vi "CreateAF-ClassLibrary.vi"(7 "Providername":string="NewActor", 8 "error in (no error)":errorcluster, 10 "ProjectTreePosition(String or Project Item Ref)":variant, 11 "CreateClassData":T1={"ClassName"="A1", "ClassFolder"=path "D:/LabVIEW/2010-T1/A1", "ClassDescription"="", "ClassTemplateOptions"="AF3.0.7_Actor1_GUI_G4_3.0.7", "BaseClass(ProjectStringPath or LvClassFilePath)"=variant(path path "C:/Program Files/National Instruments/LabVIEW 2010/user.lib/_Frameworks/Actor Framework/Actor/Actor.lvclass"), "ExtraCreateParameters"=variant, "FolderSuffix"="_Actor", "ParentInterfaces"=[]}) -> (0 "error out":errorcluster, 2 "TemplateVersionUsed":string, 3 "LVClassLibraryRefnum":refnum<vi>)   [LabVIEW 2020, in "ClassWriterNative.lvclass"]
uses:
  <resource>/Framework/Providers/Open_GDS/ClassProviders/Provider_LvNativeClass/ClassWriterNative_class/ClassWriterNative.lvclass
  <resource>/Framework/Providers/Open_GDS/ClassProviders/Provider_BaseClassInterface/CreateClassData.ctl
  <resource>/Framework/Providers/Open_GDS/ClassProviders/Common/LvClass_class/GDSLvCLass_ClassSettingsType.ctl
  <resource>/Framework/Providers/Open_GDS/ClassProviders/Common/LvClass_class/GDSLvClass_PlugIn.ctl
  <resource>/Framework/Providers/Open_GDS/ClassProviders/Common/LvClass_class/GDSLvClass_PlugInTypes.ctl
  <resource>/Framework/Providers/Open_GDS/ClassProviders/Common/ScriptingFunctions/Scripting_ConnectorPanePatternType.ctl
  <resource>/Framework/Providers/Open_GDS/ClassProviders/Provider_BaseClassInterface/ClassApperanceType.ctl
  <resource>/Framework/Providers/Open_GDS/ClassProviders/Provider_BaseClassInterface/ClassWriter_class/ClassWriter.lvclass
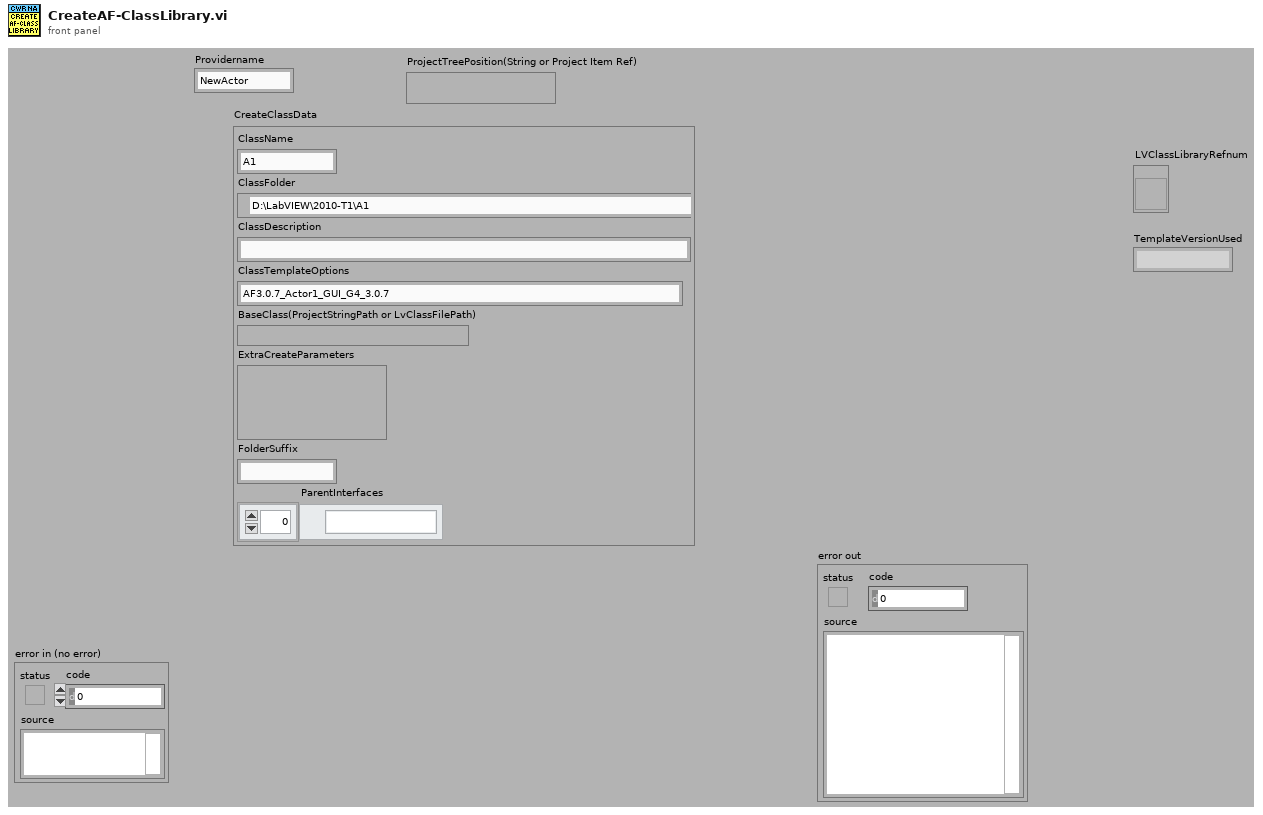
[diagram p1: front panel]
types:
  T1 = typedef "ClassWriter.lvclass/CreateClassData.ctl" = cluster{"ClassName":string, "ClassFolder":path, "ClassDescription":string, "ClassTemplateOptions":string, "BaseClass(ProjectStringPath or LvClassFilePath)":variant, "ExtraCreateParameters":variant, "FolderSuffix":string, "ParentInterfaces":path[]}
  T2 = cluster{"TemplateLib/ClassName":string, "Library":refnum<vi>, "LibraryVIs":refnum<vi>[], "LibraryClasses":refnum<vi>[], "LibraryViNames":string[], "LibraryClassesNames":string[], "TemplateLib/ClassPath":path, "ClassTemplateVersion":string, "App":refnum<vi>, "ProjectRefnum":refnum<vi>, "ProjectItemOwner":refnum<vi>, "VIsRenamed":path[], "ClassesRenamed":path[], "ClassesRootClass":string[], "lvlib":bool, "LibraryVIPaths":path[], "LibraryClassesPaths":path[], "FolderItems":refnum<vi>[], "FolderNames":string[], "AddInheritance":bool[], "LibraryClasses(Path)":path[], "DestroyProjectItemRef":bool}
  T3 = typedef "GDSLvCLass_ClassSettingsType.ctl" = cluster{"ClassProviderName":string, "ClassTemplateUsed":string, "ClassTemplateVersion":string, "ClassDescription":string, "PlugIns":T4[], "ConnectorPanePattern":string}
  T4 = typedef "GDSLvClass_PlugIn.ctl" = cluster{"Type":T5, "ID":string, "Version":string, "Path":path, "Name":string, "Data":variant}
  T5 = typedef "GDSLvClass_PlugInTypes.ctl" = enum16{"DesignPattern", "MethodTypes"}
  T6 = typedef "ClassApperanceType.ctl" = enum16{"Class", "AF-MessageClass", "Interface"}
  T7 = cluster{"LibraryIcon":string, "HeaderRows(1)":u8}
  T8 = cluster{"Major":u16, "Minor":u16, "Fix":u16, "Build":u16}
  T9 = typedef "AF_SettingsType.ctl" = cluster{"MessageFolderName":string}
  T10 = typedef "Scripting_ConnectorPanePatternType.ctl" = u16
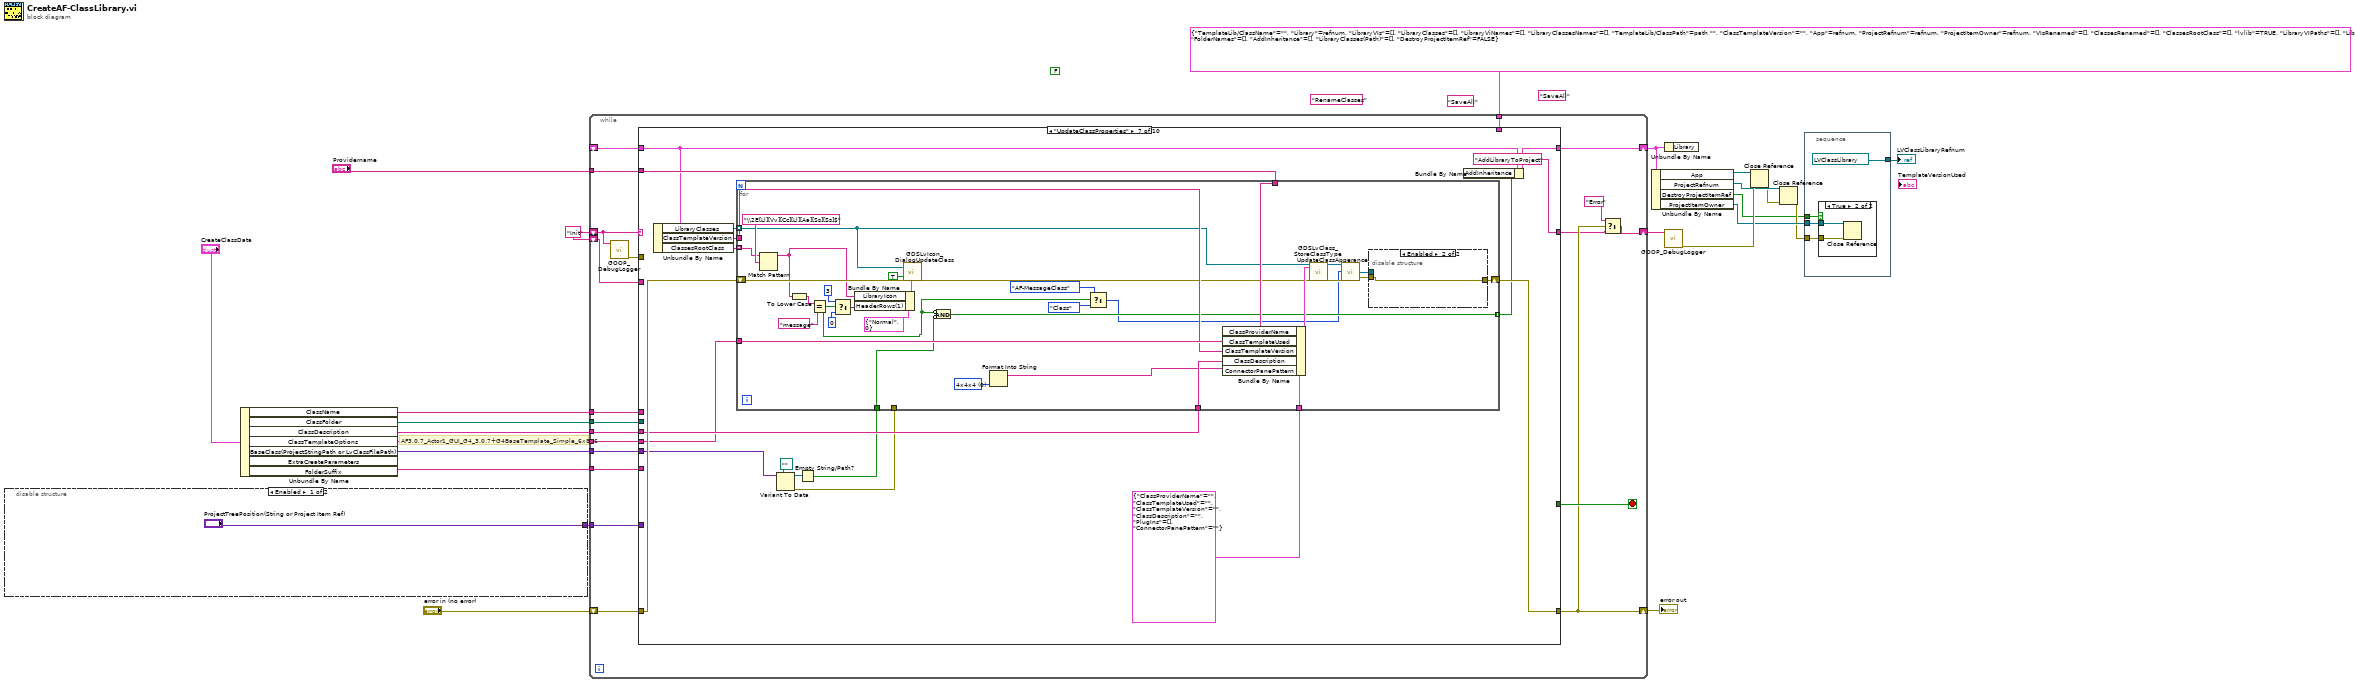
[diagram p0: block diagram]
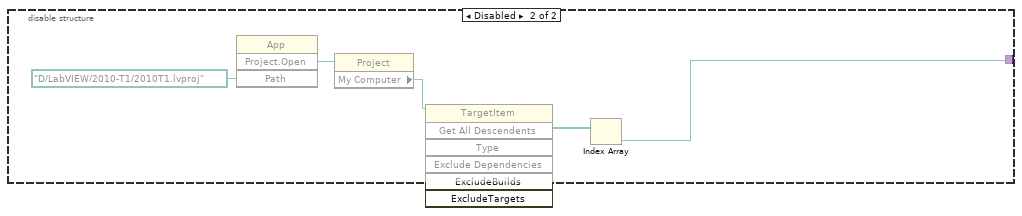
[diagram p3: hidden frame]
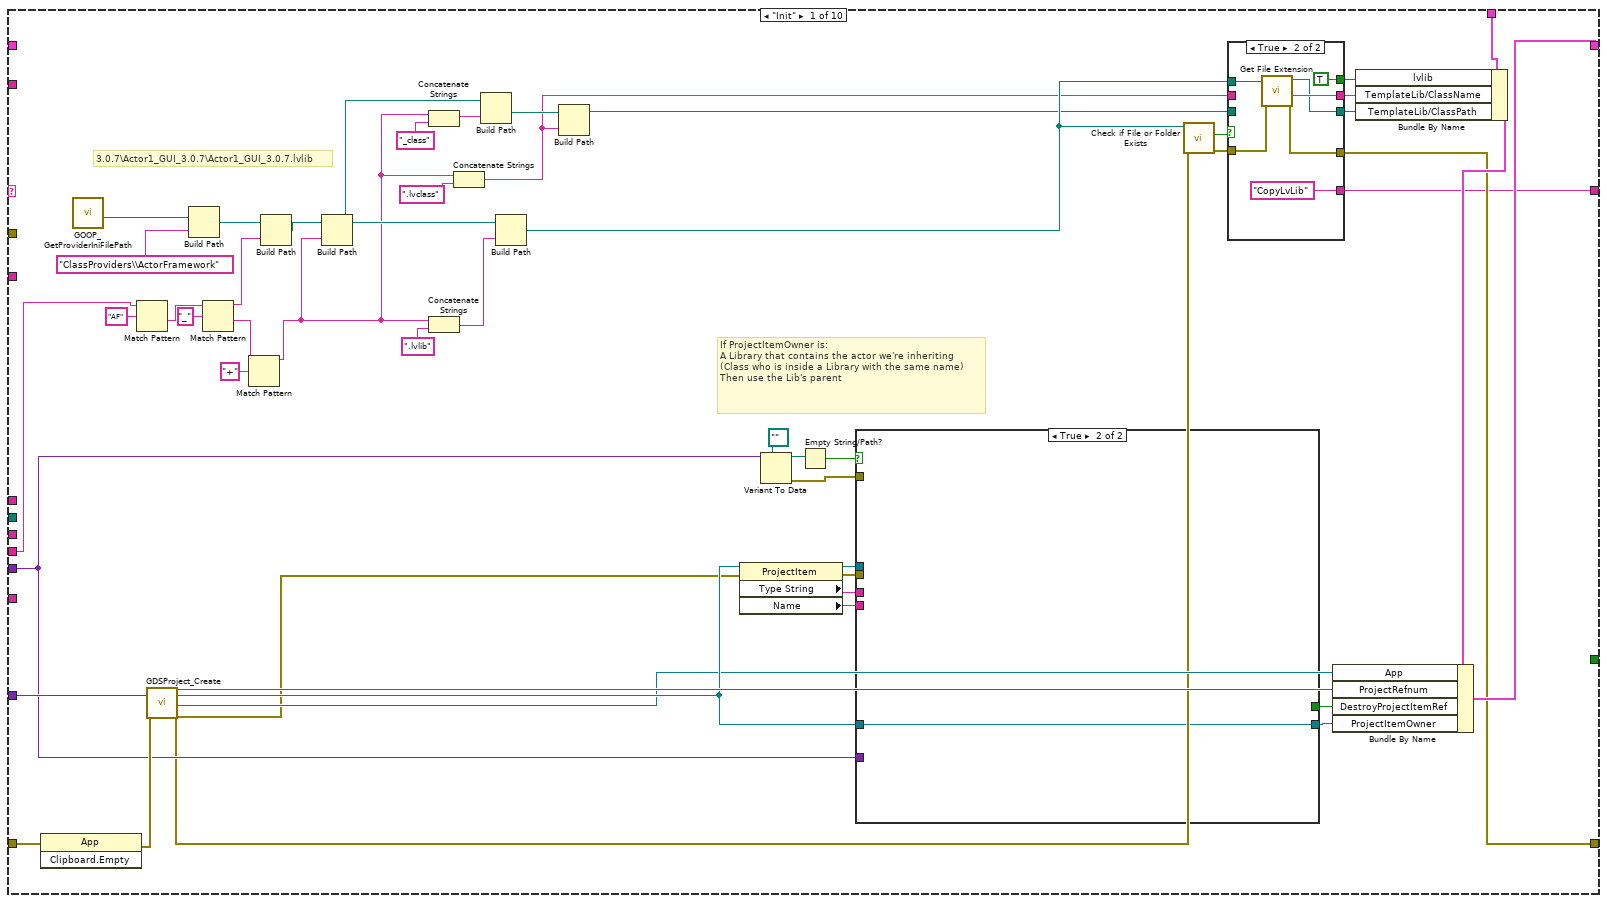
[diagram p4: hidden frame]
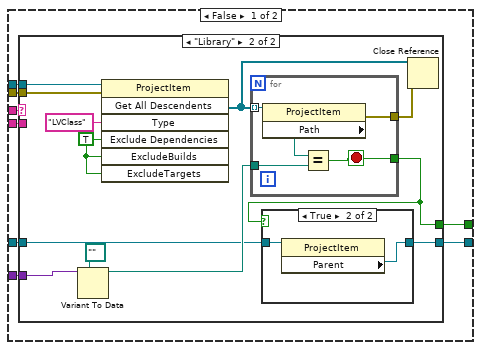
[diagram p5: hidden frame]
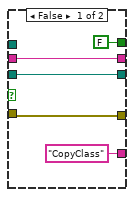
[diagram p8: hidden frame]
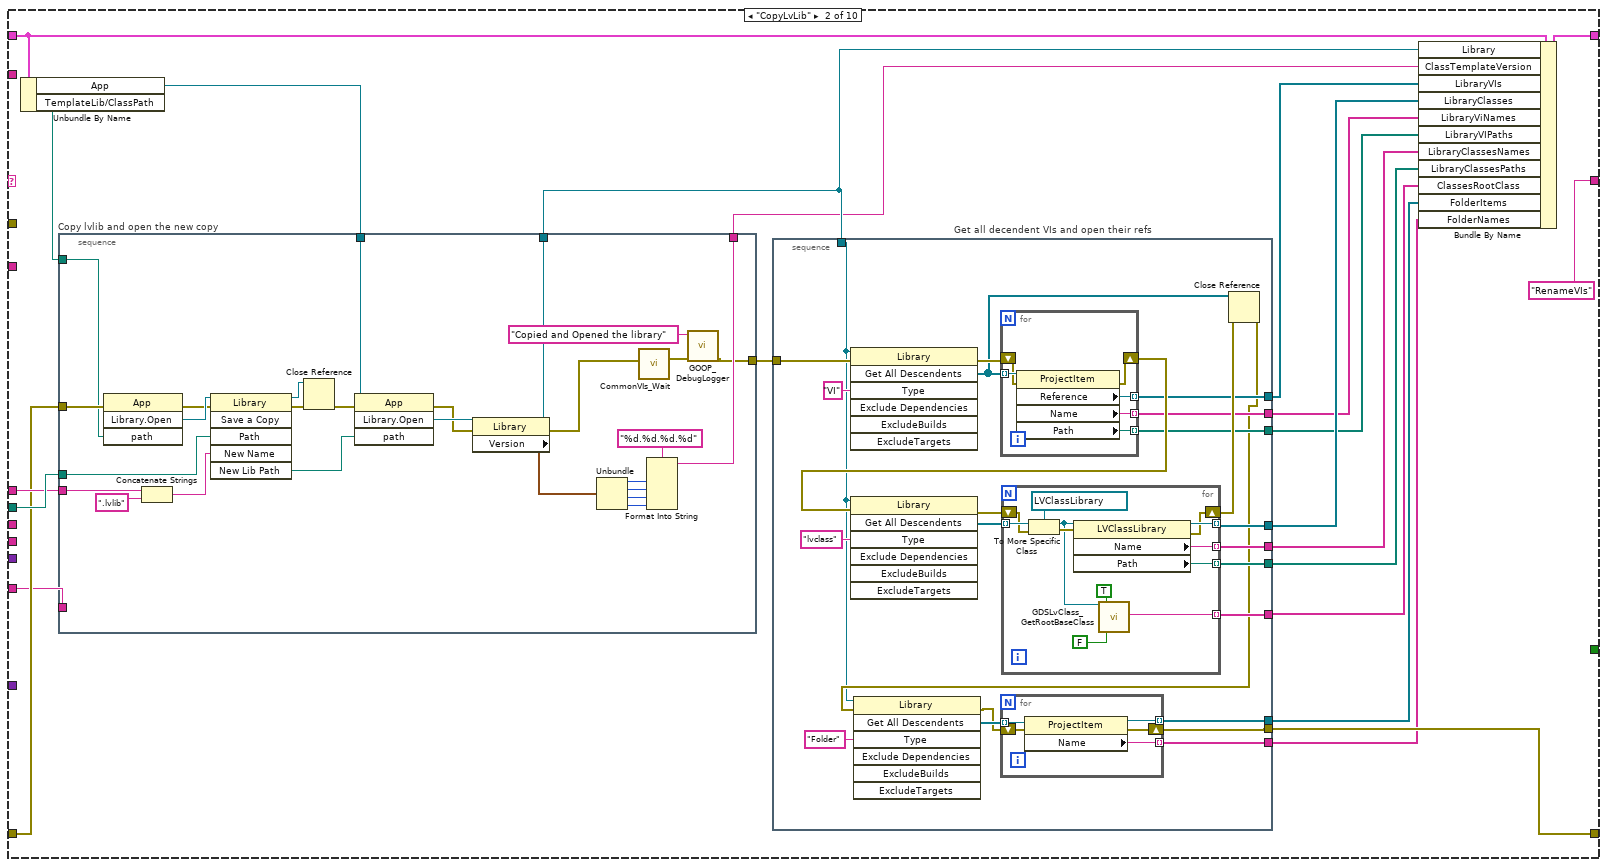
[diagram p9: hidden frame]
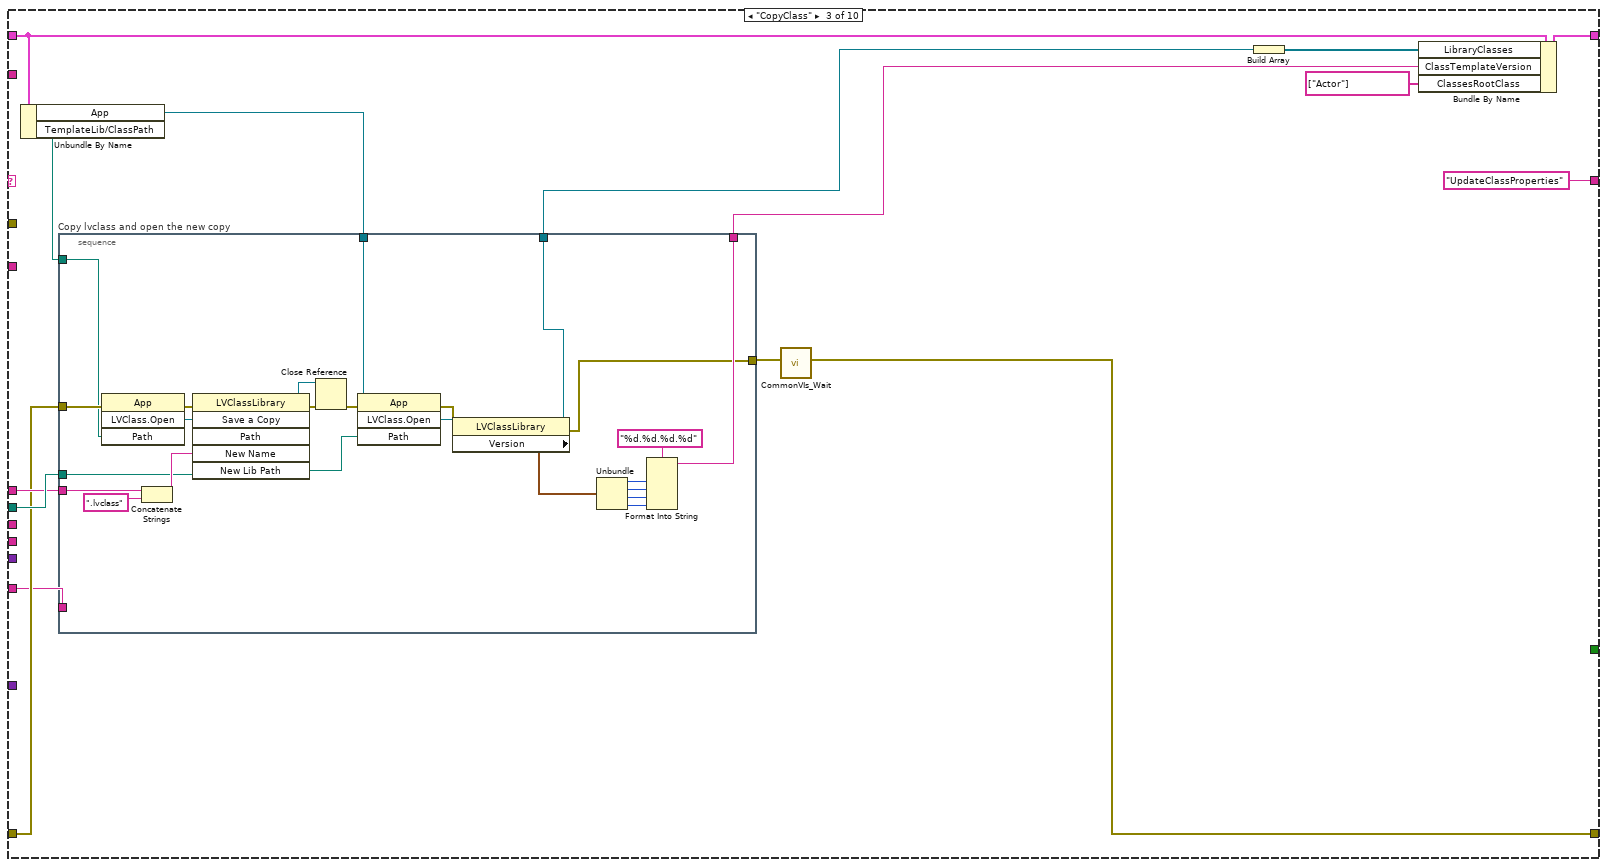
[diagram p10: hidden frame]
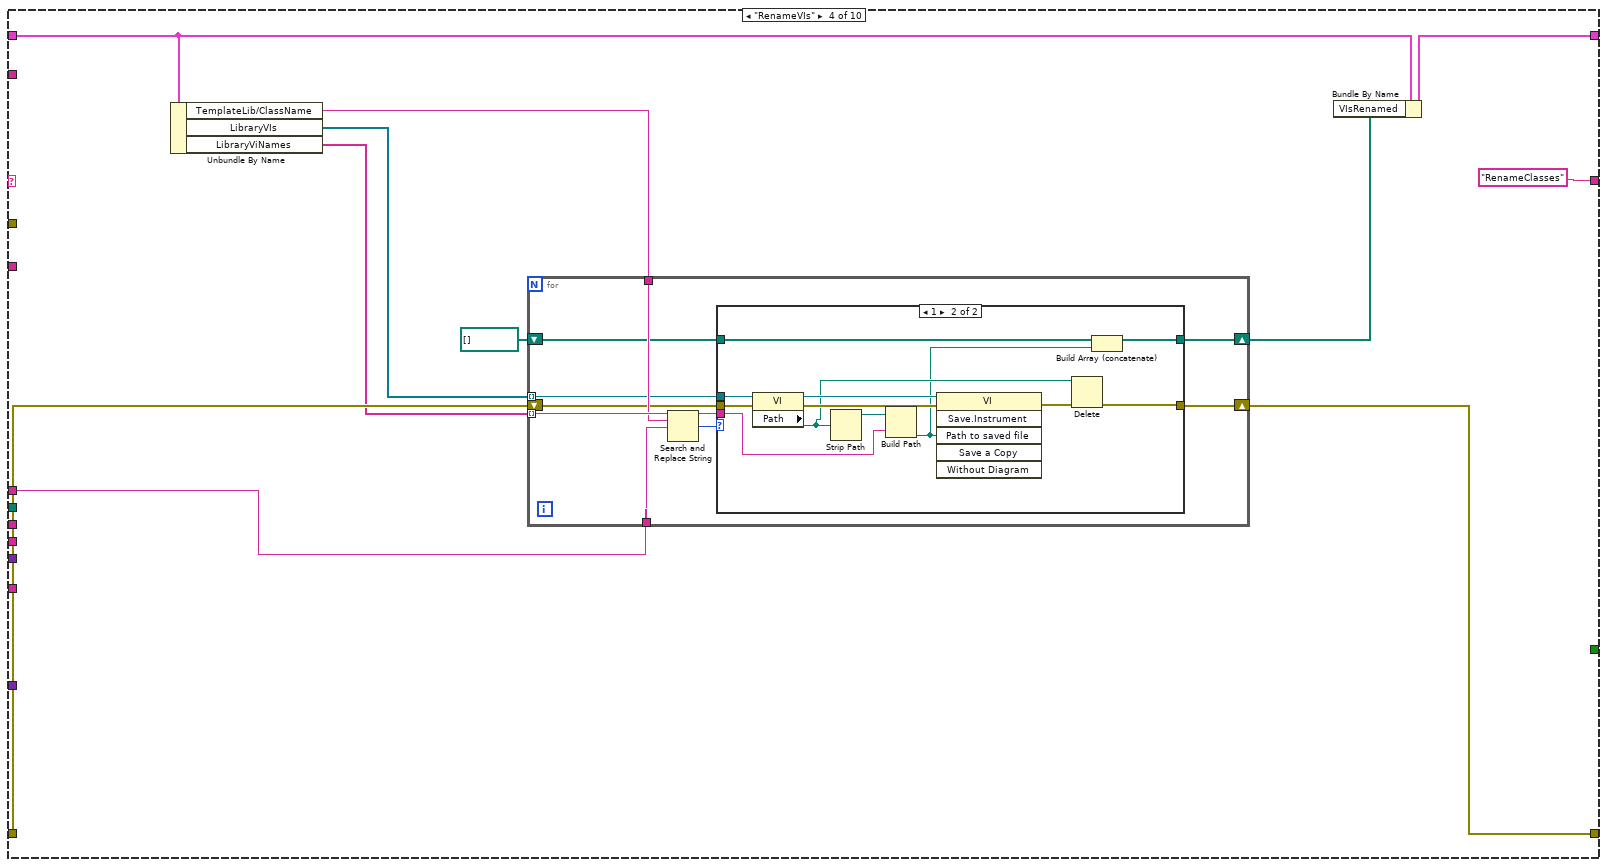
[diagram p11: hidden frame]
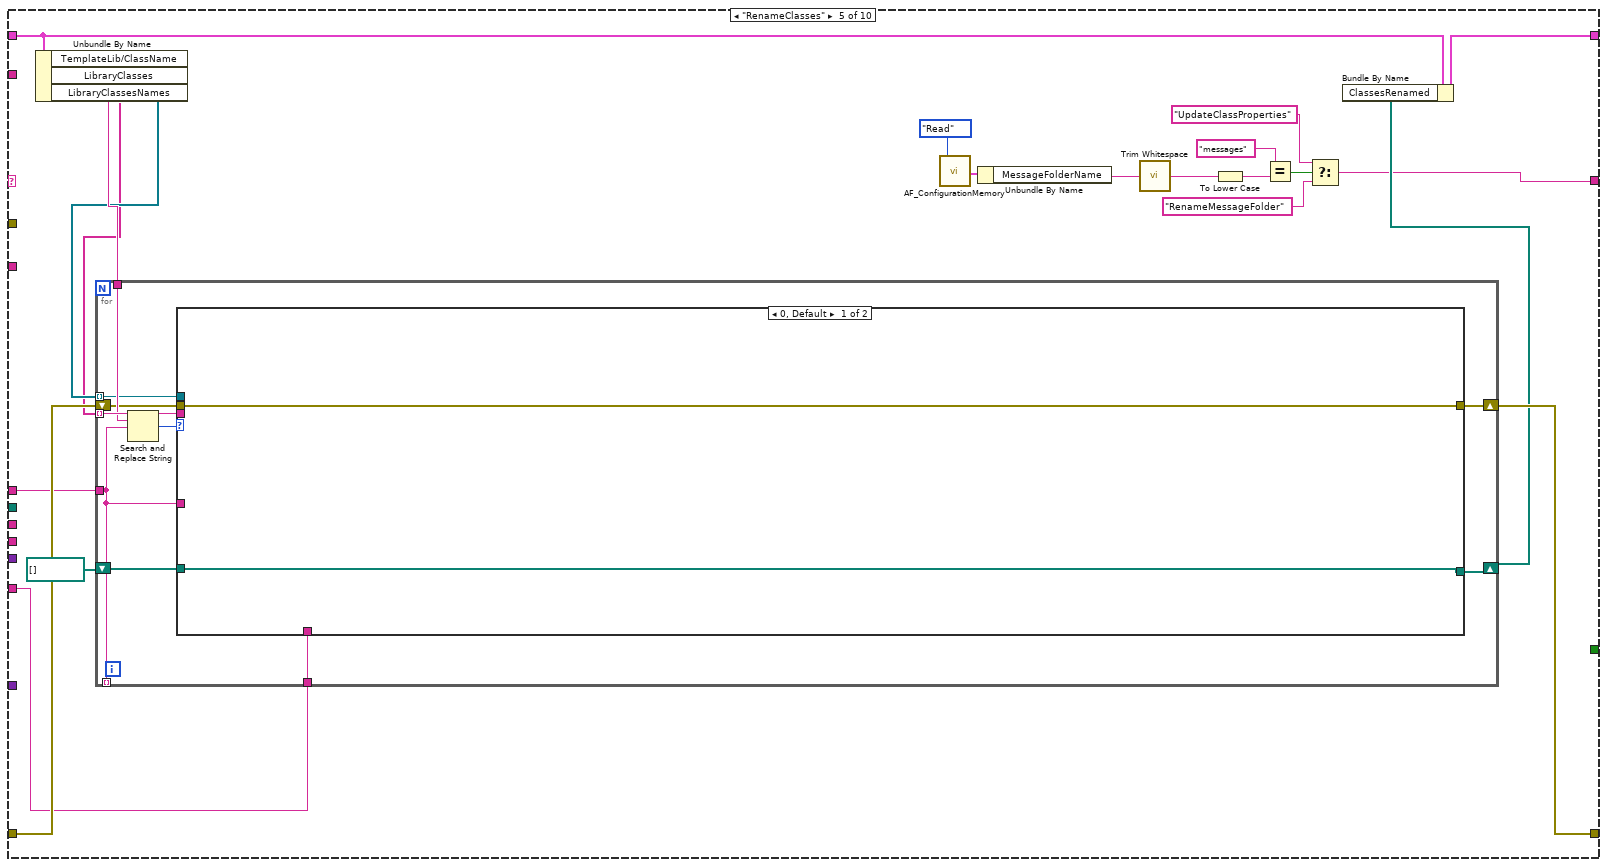
[diagram p13: hidden frame]
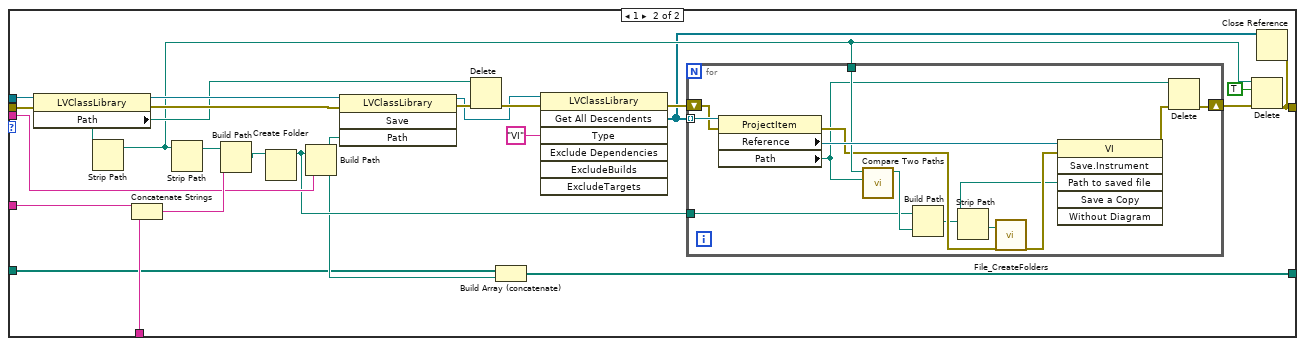
[diagram p14: hidden frame]
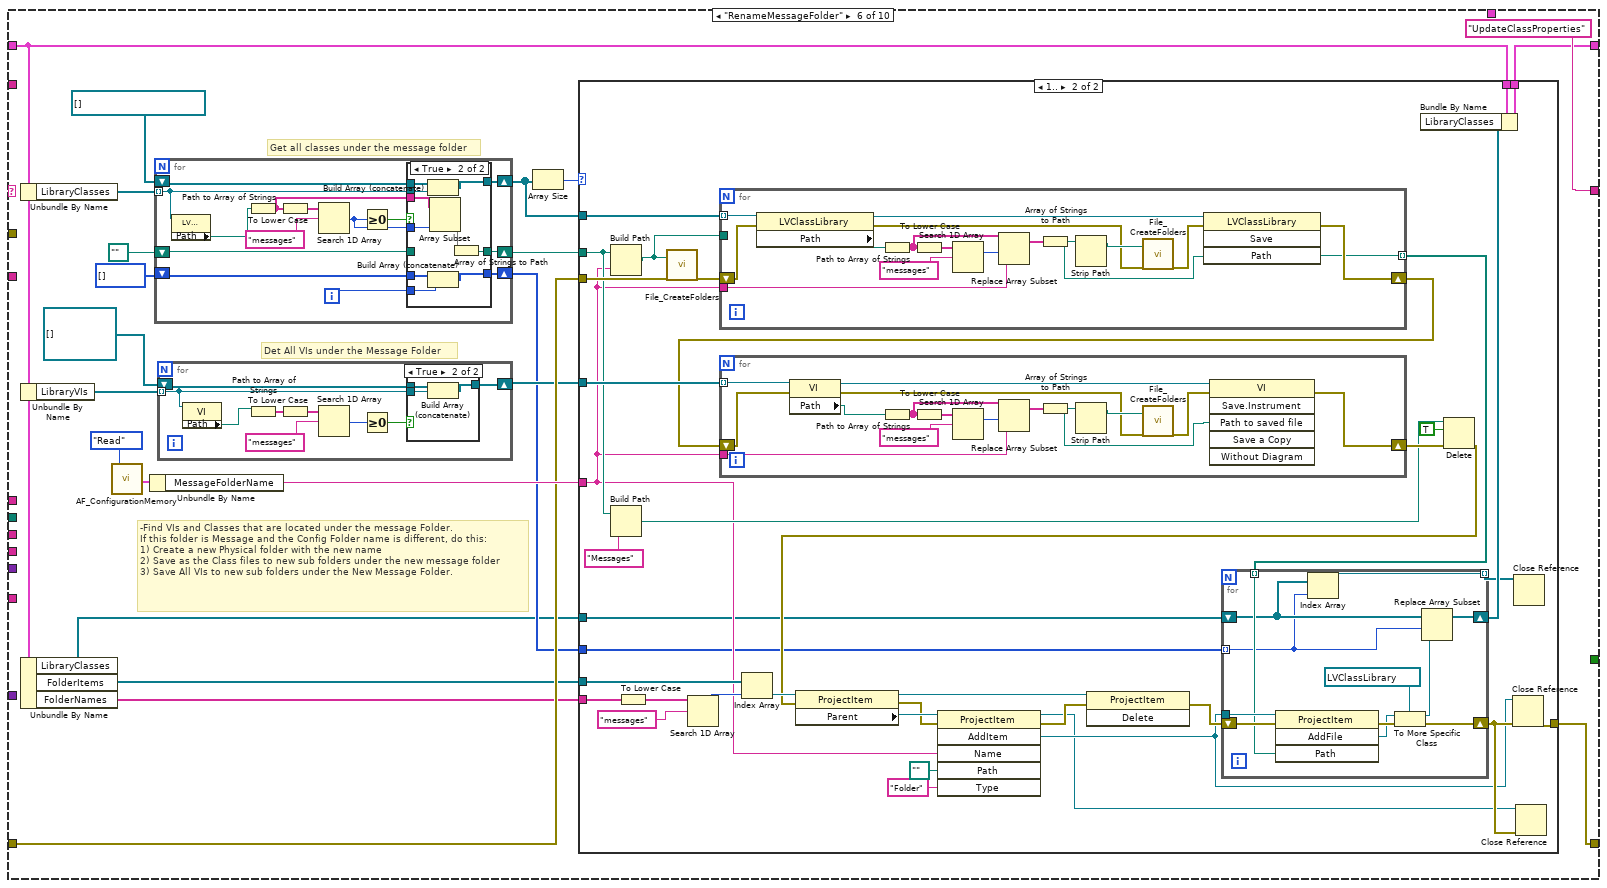
[diagram p15: hidden frame]
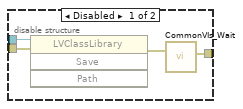
[diagram p19: hidden frame]
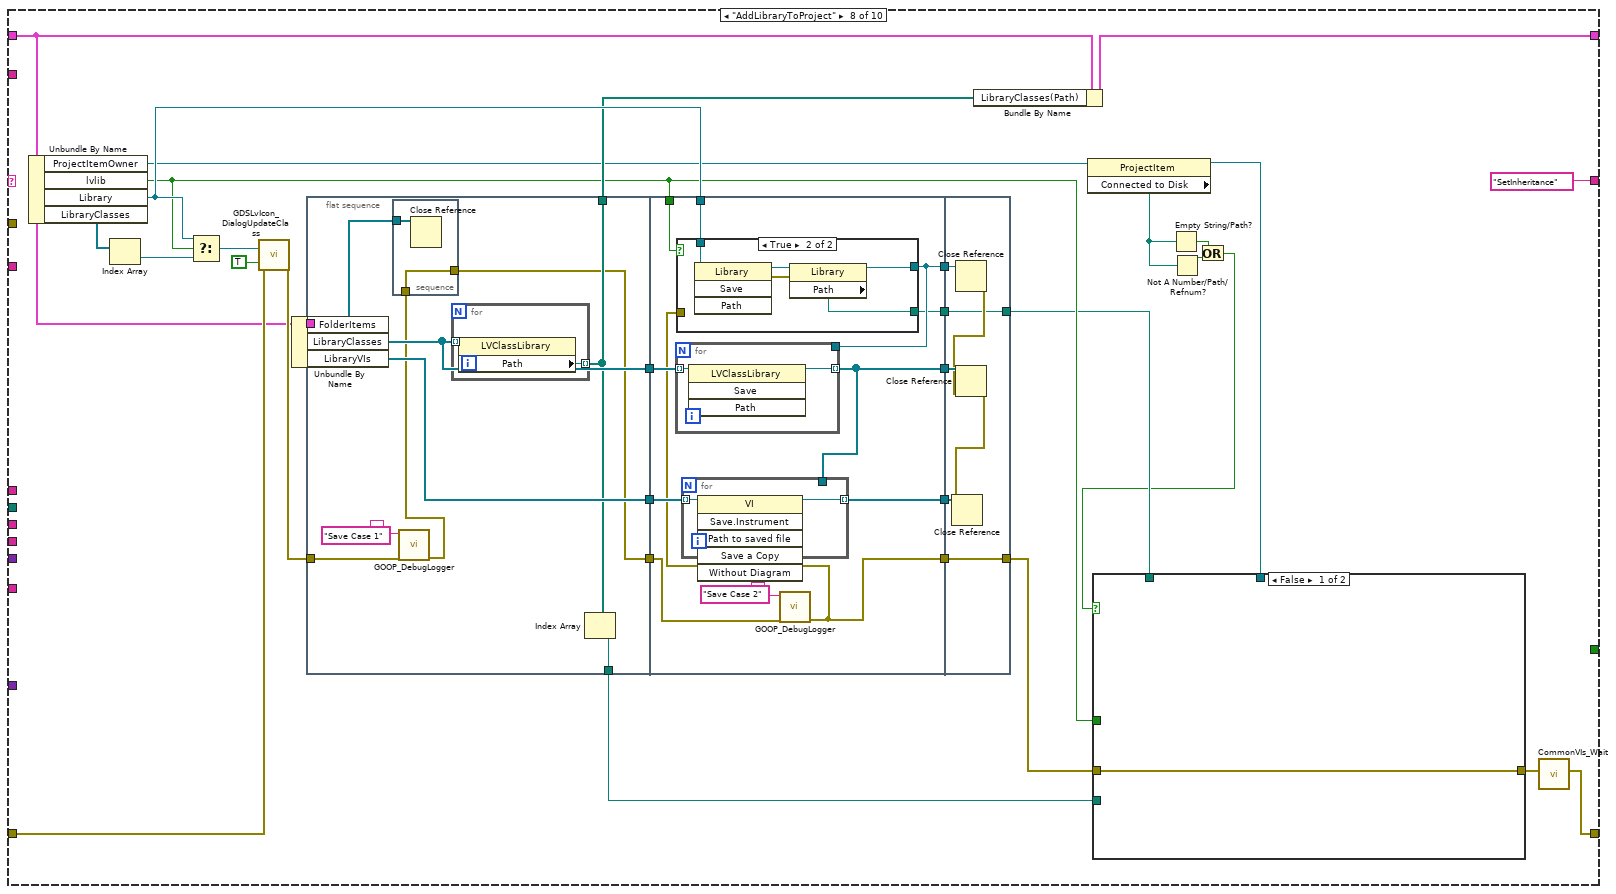
[diagram p20: hidden frame]
diagram:
  (unwired) FALSE ("LimitToSpecificProviderTypeOfSameType(True)")
  (unwired) "RenameClasses" ("Name")
  (unwired) "SaveAll" ("Name")
  (unwired) "SaveAll" ("Name")
  w1 = "Init" ("string")
  # "AF3.0.7_Actor1_GUI_G4_3.0.7+G4BaseTemplate_Simple_6x8x6"
  n1 = disable-structure shown="Enabled" {
    disable-tunnel: ["ProjectTreePosition(String or Project Item Ref)" w25] -> w13
    frame Enabled {
    }
    frame Disabled {
      n2 = invoke class="App" method="Project.Open"("Path"=path "D:/LabVIEW/2010-T1/2010T1.lvproj") -> ("Project:Open"=w28:refnum<vi>)  [unwired: 3 in, 3 out]
      n3 = property class="Project"(reference=w28) -> ("My Computer"=w26:refnum<vi>)  [unwired: 1 in, 2 out]
      n4 = invoke class="TargetItem" method="Get All Descendents"(reference=w26) -> ("All Descendents"=w27:refnum<vi>[])  [unwired: 6 in, 6 out]
      n5 = Index Array(array=w27) -> (element=w25:refnum<vi>)  [unwired: 1 in]
    }
  }
  n6 = Unbundle By Name("CreateClassData") -> ("ClassName"=w20:string, "ClassFolder"=w17:path, "ClassDescription"=w14:string, "ClassTemplateOptions"=w16:string, "BaseClass(ProjectStringPath or LvClassFilePath)"=w11:variant, "FolderSuffix"=w19:string)  [unwired: 1 out]
  n7 = while {
    tunnel: w17 -> [w49]
    tunnel: w20 -> [w48]
    tunnel: w19 -> [w46]
    shift-right: [w31] -> w9
    shift-left: w1 -> [w36]
    shift-right: [w44] -> w12
    shift-left: _ -> [w43]
    tunnel: T2 {"TemplateLib/ClassName"="", "Library"=refnum, "LibraryVIs"=[], "LibraryClasses"=[], "LibraryViNames"=[], "LibraryClassesNames"=[], "TemplateLib/ClassPath"=path "", "ClassTemplateVersion"="", "App"=refnum, "ProjectRefnum"=refnum, "ProjectItemOwner"=refnum, "VIsRenamed"=[], "ClassesRenamed"=[], "ClassesRootClass"=[], "lvlib"=TRUE, "LibraryVIPaths"=[], "LibraryClassesPaths"=[], "FolderItems"=[], "FolderNames"=[], "AddInheritance"=[], "LibraryClasses(Path)"=[], "DestroyProjectItemRef"=FALSE} -> [w45]
    shift-right: [w33] -> w18
    shift-left: "error in (no error)" -> [w47]
    tunnel: w16 -> [w41]
    tunnel: "Providername" -> [w40]
    tunnel: w14 -> [w39]
    tunnel: w13 -> [w38]
    tunnel: w11 -> [w37]
    shift-left: w1 -> [w34]
    stop <- w42 stop-if-true
    n8 = call <resource>:"GOOP_DebugLogger.vi"("State"=w36) -> ("error out"=w35:errorcluster)  [unwired: 8 in, 2 out]
    n9 = case shown="\"UpdateClassProperties\"" w36 {
      tunnel: w49 -> [_ w163 w252 _ _ _ _ _ _ _]
      tunnel: w48 -> [_ w162 w251 w284 w328 _ _ _ _ _]
      tunnel: [w78 w160 w239 w285 w326 w389 w535 w597 w686 w708] -> w33
      tunnel: w47 -> [w65 w159 w250 w286 w332 w393 w542 w612 w687 w709]
      tunnel: w46 -> [_ w158 w249 _ w327 _ _ _ _ _]
      tunnel: w45 -> [w99 _ _ _ _ _ _ _ _ _]
      tunnel: [w85 w152 w247 w278 w323 w384 w532 w593 w685 w706] -> w44
      tunnel: [w75 "RenameVIs" ("Name") "UpdateClassProperties" ("filename without extension") "RenameClasses" ("Name") w313 "UpdateClassProperties" ("filename without extension") "AddLibraryToProject" ("Name") "SetInheritance" ("Name") "Exit" ("Name") "Exit" ("Name")] -> w32
      tunnel: w43 -> [_ w149 w245 w279 w324 w385 w533 w594 w685 w706]
      tunnel: [_ _ _ _ _ _ _ _ _ TRUE] -> w42
      tunnel: w41 -> [w94 _ _ _ _ _ w538 _ _ _]
      tunnel: w40 -> [_ _ _ _ _ _ w541 _ _ _]
      tunnel: w39 -> [_ _ _ _ _ _ w540 _ _ _]
      tunnel: w38 -> [w83 _ _ _ _ _ _ _ _ _]
      tunnel: w37 -> [w56 _ _ _ _ _ w529 _ w683 _]
      tunnel: w35 -> [_ _ _ _ _ _ _ _ _ _]
      tunnel: w34 -> [_ _ _ _ _ _ _ _ _ w707]
      frame "Init" {
        # "If ProjectItemOwner is:\nA Library that contains the actor we're inheriting\n(Class who is inside a Library with the same name)\nThen use the Lib's parent"
        # "3.0.7\\Actor1_GUI_3.0.7\\Actor1_GUI_3.0.7.lvlib"
        n10 = invoke class="App" method="Clipboard.Empty"(error in=w65) -> (error out=w64:errorcluster)  [unwired: 2 in, 2 out]
        n11 = call <resource>:"GOOP_GetProviderIniFilePath.vi"() -> ("ProviderMainFolder"=w96:path)  [unwired: 10 in, 1 out]
        n12 = Match Pattern(string=w94, regular expression="AF") -> (after substring=w92:string)  [unwired: 1 in, 3 out]
        n13 = call <resource>:"GDSProject_Create.vi"("ProjectTreePosition(String or Project Item Ref)"=w83, "error in (no error)"=w64) -> ("Project Refnum"=w86:refnum<vi>, "Project Item"=w59:refnum<vi>, "App"=w51:refnum<vi>, "error out"=w50:errorcluster)  [unwired: 13 in, 1 out]
        n14 = Build Path(base path=w96, name or relative path="ClassProviders\\ActorFramework") -> (appended path=w97:path)
        n15 = Match Pattern(string=w92, regular expression="_") -> (before substring=w90:string, after substring=w82:string)  [unwired: 1 in, 2 out]
        n16 = Match Pattern(string=w82, regular expression="+") -> (before substring=w70:string)  [unwired: 1 in, 3 out]
        n17 = Build Path(base path=w97, name or relative path=w90) -> (appended path=w89:path)
        n18 = Build Path(base path=w89, name or relative path=w70) -> (appended path=w74:path)
        n19 = Concatenate Strings(w70, "_class" ("string")) -> (w72:string)
        n20 = Concatenate Strings(w70, ".lvlib" ("string")) -> (w87:string)
        n21 = Concatenate Strings(w70, ".lvclass" ("string")) -> (w68:string)
        n22 = Build Path(base path=w74, name or relative path=w72) -> (appended path=w71:path)
        n23 = Build Path(base path=w74, name or relative path=w87) -> (appended path=w80:path)
        n24 = Build Path(base path=w71, name or relative path=w68) -> (appended path=w67:path)
        n25 = property class="ProjectItem"(reference=w59, error in=w50) -> (reference out=w61:refnum<vi>, error out=w60:errorcluster, "Type String"=w63:string, "Name"=w62:string)
        n26 = Variant To Data(type=path "" ("Path"), Variant=w56) -> (data=w54:path, error out=w52:errorcluster)  [unwired: 1 in]
        n27 = Empty String/Path?(string/path=w54) -> (empty?=w53:bool)
        n28 = case shown="True" w53 {
          tunnel: w63 -> [w107 _]
          tunnel: w62 -> [w106 _]
          tunnel: w61 -> [w105 _]
          tunnel: w60 -> [w104 _]
          tunnel: w56 -> [w103 _]
          tunnel: w59 -> [w102 w129]
          tunnel: [w101 w129] -> w58
          tunnel: [w100 _] -> w57
          tunnel: w52 -> [_ _]
          frame False {
            n29 = case shown="\"Library\"" w107 {
              tunnel: w106 -> [_ _]
              tunnel: w105 -> [_ w120]
              tunnel: w104 -> [_ w119]
              tunnel: w103 -> [_ w116]
              tunnel: w102 -> [w108 w113]
              tunnel: [w108 w112] -> w101
              tunnel: [_ w111] -> w100
              frame "False", Default {
              }
              frame "Library" {
                w117 = TRUE ("ExcludeDependencies")
                n30 = Variant To Data(type=path "" ("Path"), Variant=w116) -> (data=w115:path)  [unwired: 1 in, 1 out]
                n31 = invoke class="ProjectItem" method="Get All Descendents"(reference=w120, error in=w119, "Type"="LVClass", "Exclude Dependencies"=w117, "ExcludeBuilds"=w117, "ExcludeTargets"=w117) -> ("All Descendents"=w109:refnum<vi>[])  [unwired: 1 in, 6 out]
                n32 = for {
                  tunnel: w109 -> [w128] mode=indexing
                  tunnel: w115 -> [w126]
                  tunnel: [w125] -> w111
                  tunnel: [w124] -> w110
                  stop <- w125 stop-if-true
                  n33 = property class="ProjectItem"(reference=w128) -> (error out=w124:errorcluster, "Path"=w127:path)  [unwired: 1 in, 1 out]
                  n34 = Equal?(x=w127, y=w126) -> (x = y?=w125:bool)
                }
                n35 = case shown="True" w111 {
                  tunnel: w113 -> [w121 w123]
                  tunnel: [w121 w122] -> w112
                  frame False {
                  }
                  frame True {
                    n36 = property class="ProjectItem"(reference=w123) -> ("Parent"=w122:refnum<vi>)  [unwired: 1 in, 2 out]
                  }
                }
                n37 = Close Reference(reference=w109, error in (no error)=w110) -> ()  [unwired: 1 out]
              }
            }
          }
          frame True {
          }
        }
        n38 = call <vilib>:"Check if File or Folder Exists.vi"("error in (no error)"=w50, "path"=w80) -> ("error out"=w79:errorcluster, "file or folder exists?"=w77:bool)  [unwired: 7 in, 1 out]
        n39 = case shown="True" w77 {
          tunnel: [w132 w141] -> w98
          tunnel: w80 -> [_ w140]
          tunnel: w79 -> [w134 w139]
          tunnel: [w134 w138] -> w78
          tunnel: [w131 w137] -> w76
          tunnel: ["CopyClass" ("Name") "CopyLvLib" ("Name")] -> w75
          tunnel: w68 -> [w132 _]
          tunnel: w67 -> [w131 _]
          tunnel: [FALSE TRUE] -> w66
          frame False {
          }
          frame True {
            n40 = call <vilib>:"Get File Extension.vi"("error in (no error)"=w139, "file"=w140) -> ("error out"=w138:errorcluster, "filename without extension"=w141:string, "dup file"=w137:path)  [unwired: 5 in, 2 out]
          }
        }
        n41 = Bundle By Name(cluster=w99, "lvlib"=w66, "TemplateLib/ClassName"=w98, "TemplateLib/ClassPath"=w76) -> (w84:T2)
        n42 = Bundle By Name(cluster=w84, "App"=w51, "ProjectRefnum"=w86, "DestroyProjectItemRef"=w57, "ProjectItemOwner"=w58) -> (w85:T2)
      }
      frame "CopyLvLib" {
        n43 = Unbundle By Name(w149) -> ("App"=w142:refnum<vi>, "TemplateLib/ClassPath"=w150:path)
        n44 = stacked-sequence "Copy lvlib and open the new copy" {
          tunnel: w163 -> [w226]
          tunnel: w158 -> [_]
          tunnel: w162 -> [w233]
          tunnel: [w217] -> w157
          tunnel: [w213] -> w161
          tunnel: w159 -> [w228]
          tunnel: w150 -> [w227]
          tunnel: [w216] -> w148
          tunnel: w142 -> [w211]
          frame #0 {
            n45 = invoke class="App" method="Library.Open"(error in=w228, "path"=w227) -> (error out=w235:errorcluster, "Open Library"=w237:refnum<vi>)  [unwired: 2 in, 2 out]
            n46 = Concatenate Strings(w233, ".lvlib" ("string")) -> (w236:string)
            n47 = invoke class="Library" method="Save a Copy"(reference=w237, error in=w235, "Path"=w226, "New Name"=w236) -> (reference out=w230:refnum<vi>, error out=w232:errorcluster, "New Lib Path"=w229:path)  [unwired: 2 in, 3 out]
            n48 = Close Reference(reference=w230, error in (no error)=w232) -> (error out=w231:errorcluster)
            n49 = invoke class="App" method="Library.Open"(reference=w211, error in=w231, "path"=w229) -> (error out=w218:errorcluster, "Open Library"=w219:refnum<vi>)  [unwired: 1 in, 2 out]
            n50 = property class="Library"(reference=w219, error in=w218) -> (reference out=w217:refnum<vi>, error out=w215:errorcluster, "Version"=w220:T8)
            n51 = Unbundle(w220) -> ("Major"=w222:u16, "Minor"=w223:u16, "Fix"=w224:u16, "Build"=w225:u16)
            n52 = call <resource>:"CommonVIs_Wait.vi"("error in"=w215) -> ("error out"=w214:errorcluster)  [unwired: 9 in]
            n53 = Format Into String(format string="%d.%d.%d.%d", w222, w223, w224, w225) -> (resulting string=w216:string)  [unwired: 2 in, 1 out]
            n54 = call <resource>:"GOOP_DebugLogger.vi"("error in (no error)"=w214, "State"="Copied and Opened the library") -> ("error out"=w213:errorcluster)  [unwired: 7 in, 2 out]
          }
        }
        n55 = stacked-sequence "Get all decendent VIs and open their refs" {
          tunnel: w157 -> [w170]
          tunnel: w161 -> [w187]
          tunnel: [w166] -> w160
          tunnel: [w178] -> w156
          tunnel: [w177] -> w153
          tunnel: [w176] -> w154
          tunnel: [w175] -> w155
          tunnel: [w174] -> w147
          tunnel: [w173] -> w146
          tunnel: [w172] -> w145
          tunnel: [w167] -> w144
          tunnel: [w164] -> w143
          frame #0 {
            n56 = invoke class="Library" method="Get All Descendents"(reference=w170, error in=w187, "Type"="VI") -> (error out=w185:errorcluster, "All Descendents"=w184:refnum<vi>[])  [unwired: 4 in, 5 out]
            n57 = for {
              tunnel: w184 -> [w210] mode=indexing
              shift-right: [w208] -> w182
              shift-left: w185 -> [w209]
              tunnel: [w207] -> w178 mode=indexing
              tunnel: [w206] -> w176 mode=indexing
              tunnel: [w205] -> w173 mode=indexing
              n58 = property class="ProjectItem"(reference=w210, error in=w209) -> (error out=w208:errorcluster, "Reference"=w207:refnum<vi>, "Name"=w206:string, "Path"=w205:path)  [unwired: 1 out]
            }
            n59 = invoke class="Library" method="Get All Descendents"(reference=w170, error in=w182, "Type"="lvclass") -> (error out=w180:errorcluster, "All Descendents"=w181:refnum<vi>[])  [unwired: 4 in, 5 out]
            n60 = for {
              tunnel: w181 -> [w204] mode=indexing
              shift-right: [w200] -> w179
              shift-left: w180 -> [w202]
              tunnel: [w201] -> w175 mode=indexing
              tunnel: [w198] -> w177 mode=indexing
              tunnel: [w194] -> w174 mode=indexing
              tunnel: [w193] -> w172 mode=indexing
              n61 = To More Specific Class(target class=refnum<vi> refnum ("Library"), reference=w204, error in=w202) -> (specific class reference=w197:refnum<vi>, error out=w199:errorcluster)
              n62 = property class="LVClassLibrary"(reference=w197, error in=w199) -> (reference out=w201:refnum<vi>, error out=w200:errorcluster, "Name"=w198:string, "Path"=w193:path)
              n63 = call <resource>:"GDSLvClass_GetRootBaseClass.vi"("ViRef/Path,LvClassRef/Path"=w197, "Don'tOpenReference"=TRUE, "LimitToSpecificProviderTypeOfSameType(True)"=FALSE) -> ("ClassName"=w194:string)  [unwired: 10 in, 6 out]
            }
            n64 = Close Reference(reference=w184, error in (no error)=w179) -> (error out=w171:errorcluster)
            n65 = invoke class="Library" method="Get All Descendents"(reference=w170, error in=w171, "Type"="Folder") -> (error out=w165:errorcluster, "All Descendents"=w168:refnum<vi>[])  [unwired: 4 in, 5 out]
            n66 = for {
              tunnel: w168 -> [w192] mode=indexing
              tunnel: [w191] -> w167 mode=indexing
              shift-right: [w190] -> w166
              shift-left: w165 -> [w189]
              tunnel: [w188] -> w164 mode=indexing
              n67 = property class="ProjectItem"(reference=w192, error in=w189) -> (reference out=w191:refnum<vi>, error out=w190:errorcluster, "Name"=w188:string)
            }
          }
        }
        n68 = Bundle By Name(cluster=w149, "Library"=w157, "ClassTemplateVersion"=w148, "LibraryVIs"=w156, "LibraryClasses"=w155, "LibraryViNames"=w154, "LibraryVIPaths"=w146, "LibraryClassesNames"=w153, "LibraryClassesPaths"=w145, "ClassesRootClass"=w147, "FolderItems"=w144, "FolderNames"=w143) -> (w152:T2)
      }
      frame "CopyClass" {
        n69 = Unbundle By Name(w245) -> ("App"=w238:refnum<vi>, "TemplateLib/ClassPath"=w246:path)
        n70 = stacked-sequence "Copy lvclass and open the new copy" {
          tunnel: w252 -> [w265]
          tunnel: w249 -> [_]
          tunnel: w251 -> [w272]
          tunnel: [w256] -> w248
          tunnel: [w254] -> w240
          tunnel: w250 -> [w267]
          tunnel: w246 -> [w266]
          tunnel: [w255] -> w244
          tunnel: w238 -> [w253]
          frame #0 {
            n71 = invoke class="App" method="LVClass.Open"(error in=w267, "Path"=w266) -> (error out=w274:errorcluster, "LVClass.Open"=w276:refnum<vi>)  [unwired: 2 in, 2 out]
            n72 = Concatenate Strings(w272, ".lvclass" ("string")) -> (w275:string)
            n73 = invoke class="LVClassLibrary" method="Save a Copy"(reference=w276, error in=w274, "Path"=w265, "New Name"=w275) -> (reference out=w269:refnum<vi>, error out=w271:errorcluster, "New Lib Path"=w268:path)  [unwired: 2 in, 3 out]
            n74 = Close Reference(reference=w269, error in (no error)=w271) -> (error out=w270:errorcluster)
            n75 = invoke class="App" method="LVClass.Open"(reference=w253, error in=w270, "Path"=w268) -> (error out=w257:errorcluster, "LVClass.Open"=w258:refnum<vi>)  [unwired: 1 in, 2 out]
            n76 = property class="LVClassLibrary"(reference=w258, error in=w257) -> (reference out=w256:refnum<vi>, error out=w254:errorcluster, "Version"=w259:T8)
            n77 = Unbundle(w259) -> ("Major"=w261:u16, "Minor"=w262:u16, "Fix"=w263:u16, "Build"=w264:u16)
            n78 = Format Into String(format string="%d.%d.%d.%d", w261, w262, w263, w264) -> (resulting string=w255:string)  [unwired: 2 in, 1 out]
          }
        }
        n79 = call <resource>:"CommonVIs_Wait.vi"("error in"=w240) -> ("error out"=w239:errorcluster)  [unwired: 9 in]
        n80 = Build Array(w248) -> (w242:refnum<vi>[])
        n81 = Bundle By Name(cluster=w245, "LibraryClasses"=w242, "ClassTemplateVersion"=w244, "ClassesRootClass"=string[] ["Actor"]) -> (w247:T2)
      }
      frame "RenameVIs" {
        n82 = Unbundle By Name(w279) -> ("TemplateLib/ClassName"=w287:string, "LibraryVIs"=w283:refnum<vi>[], "LibraryViNames"=w282:string[])
        n83 = for {
          tunnel: w283 -> [w293] mode=indexing
          tunnel: w282 -> [w297] mode=indexing
          tunnel: w287 -> [w296]
          tunnel: w284 -> [w295]
          shift-right: [w290] -> w285
          shift-left: w286 -> [w291]
          shift-right: [w289] -> w277
          shift-left: path[] [] -> [w288]
          n84 = Search and Replace String(input string=w297, search string=w296, replace string=w295) -> (result string=w292:string, number of replacements=w294:i32)  [unwired: 5 in, 2 out]
          n85 = case shown="1" w294 {
            tunnel: w293 -> [_ w311]
            tunnel: w292 -> [_ w309]
            tunnel: w291 -> [w299 w306]
            tunnel: [w299 w304] -> w290
            tunnel: [w298 w302] -> w289
            tunnel: w288 -> [w298 w301]
            frame 0, Default {
            }
            frame 1 {
              n86 = property class="VI"(reference=w311, error in=w306) -> (reference out=w308:refnum<vi>, error out=w307:errorcluster, "Path"=w303:path)
              n87 = Strip Path(path=w303) -> (stripped path=w310:path)  [unwired: 1 out]
              n88 = Build Path(base path=w310, name or relative path=w309) -> (appended path=w300:path)
              n89 = invoke class="VI" method="Save.Instrument"(reference=w308, error in=w307, "Path to saved file"=w300) -> (error out=w305:errorcluster)  [unwired: 3 in, 5 out]
              n90 = Delete(path (use dialog)=w303, error in=w305) -> (error out=w304:errorcluster)  [unwired: 3 in, 2 out]
              n91 = Build Array (concatenate)(w301, w300) -> (w302:path[])
            }
          }
        }
        n92 = Bundle By Name(cluster=w279, "VIsRenamed"=w277) -> (w278:T2)
      }
      frame "RenameClasses" {
        n93 = Unbundle By Name(w324) -> ("TemplateLib/ClassName"=w331:string, "LibraryClasses"=w330:refnum<vi>[], "LibraryClassesNames"=w329:string[])
        n94 = for {
          tunnel: w330 -> [w340] mode=indexing
          tunnel: w329 -> [w343] mode=indexing
          tunnel: w331 -> [w342]
          tunnel: [w335] -> _ mode=indexing
          shift-right: [w336] -> w326
          shift-left: w332 -> [w338]
          tunnel: w327 -> [w337]
          tunnel: w328 -> [w335]
          shift-right: [w333] -> w322
          shift-left: path[] [] -> [w334]
          n95 = Search and Replace String(input string=w343, search string=w342, replace string=w335) -> (result string=w339:string, number of replacements=w341:i32)  [unwired: 5 in, 2 out]
          n96 = case shown="0, Default" w341 {
            tunnel: w340 -> [_ w370]
            tunnel: w339 -> [_ w362]
            tunnel: w338 -> [w345 w369]
            tunnel: [w345 w347] -> w336
            tunnel: w337 -> [_ w367]
            tunnel: w335 -> [_ w361]
            tunnel: w334 -> [w344 w349]
            tunnel: [w344 w348] -> w333
            frame 0, Default {
            }
            frame 1 {
              n97 = property class="LVClassLibrary"(reference=w370, error in=w369) -> (reference out=w364:refnum<vi>, error out=w363:errorcluster, "Path"=w359:path)
              n98 = Strip Path(path=w359) -> (stripped path=w353:path)  [unwired: 1 out]
              n99 = Concatenate Strings(w361, w367) -> (w366:string)
              n100 = Strip Path(path=w353) -> (stripped path=w368:path)  [unwired: 1 out]
              n101 = Build Path(base path=w368, name or relative path=w366) -> (appended path=w365:path)
              n102 = Create Folder(path (use dialog)=w365) -> (created path=w352:path)  [unwired: 2 in, 2 out]
              n103 = Build Path(base path=w352, name or relative path=w362) -> (appended path=w350:path)
              n104 = invoke class="LVClassLibrary" method="Save"(reference=w364, error in=w363, "Path"=w350) -> (reference out=w357:refnum<vi>, error out=w360:errorcluster)  [unwired: 1 in, 2 out]
              n105 = Delete(path (use dialog)=w359, error in=w360) -> (error out=w358:errorcluster)  [unwired: 3 in, 2 out]
              n106 = Build Array (concatenate)(w349, w350) -> (w348:path[])
              n107 = invoke class="LVClassLibrary" method="Get All Descendents"(reference=w357, error in=w358, "Type"="VI") -> (error out=w354:errorcluster, "All Descendents"=w346:refnum<vi>[])  [unwired: 4 in, 5 out]
              n108 = for {
                tunnel: w346 -> [w383] mode=indexing
                tunnel: w353 -> [w380]
                tunnel: w352 -> [w378]
                shift-right: [w372] -> w351
                shift-left: w354 -> [w382]
                n109 = property class="ProjectItem"(reference=w383, error in=w382) -> (error out=w377:errorcluster, "Reference"=w381:refnum<vi>, "Path"=w371:path)  [unwired: 1 out]
                n110 = call <vilib>:"Compare Two Paths.vi"("Path 2"=w371, "Path 1"=w380) -> ("Relative Path from 1 to 2"=w379:path)  [unwired: 6 in, 3 out]
                n111 = Build Path(base path=w378, name or relative path=w379) -> (appended path=w374:path)
                n112 = Strip Path(path=w374) -> (stripped path=w375:path)  [unwired: 1 out]
                n113 = call <resource>:"File_CreateFolders.vi"("Path"=w375, "error in (no error)"=w377) -> ("error out"=w376:errorcluster)  [unwired: 15 in, 2 out]
                n114 = invoke class="VI" method="Save.Instrument"(reference=w381, error in=w376, "Path to saved file"=w374) -> (error out=w373:errorcluster)  [unwired: 3 in, 5 out]
                n115 = Delete(path (use dialog)=w371, error in=w373) -> (error out=w372:errorcluster)  [unwired: 3 in, 2 out]
              }
              n116 = Delete(path (use dialog)=w353, entire hierarchy (F)=TRUE, error in=w351) -> (error out=w347:errorcluster)  [unwired: 2 in, 2 out]
              n117 = Close Reference(reference=w346, error in (no error)=w347) -> ()  [unwired: 1 out]
            }
          }
        }
        n118 = call <resource>:"AF_ConfigurationMemory.vi"("Action"=enum16{"Read", "Load", "Save", "Set"}."Read") -> ("AF_SettingsOut"=w320:T9)  [unwired: 15 in, 3 out]
        n119 = Unbundle By Name(w320) -> ("MessageFolderName"=w319:string)
        n120 = call <vilib>:"Trim Whitespace.vi"("string"=w319) -> ("trimmed string"=w312:string)  [unwired: 1 in]
        n121 = To Lower Case(string=w312) -> (all lower case string=w318:string)
        n122 = Equal?(x="messages", y=w318) -> (x = y?=w316:bool)
        n123 = Select(t="UpdateClassProperties" ("filename without extension"), s=w316, f="RenameMessageFolder" ("filename without extension")) -> (s? t:f=w313:string)
        n124 = Bundle By Name(cluster=w324, "ClassesRenamed"=w322) -> (w323:T2)
      }
      frame "RenameMessageFolder" {
        # "Det All VIs under the Message Folder"
        # "Get all classes under the message folder"
        # "-Find VIs and Classes that are located under the message Folder.\nIf this folder is Message and the Config Folder name is different, do this:\n1) Create a new Physical folder with the new name\n2) Save as the Class files to new sub folders under the new message folder\n3) Save All VIs to new sub folders under the New Message Folder."
        n125 = Unbundle By Name(w385) -> ("LibraryClasses"=w404:refnum<vi>[])
        n126 = Unbundle By Name(w385) -> ("LibraryVIs"=w402:refnum<vi>[])
        n127 = Unbundle By Name(w385) -> ("LibraryClasses"=w386:refnum<vi>[], "FolderItems"=w390:refnum<vi>[], "FolderNames"=w391:string[])
        n128 = call <resource>:"AF_ConfigurationMemory.vi"("Action"=enum16{"Read", "Load", "Save", "Set"}."Read") -> ("AF_SettingsOut"=w399:T9)  [unwired: 15 in, 3 out]
        n129 = Unbundle By Name(w399) -> ("MessageFolderName"=w395:string)
        n130 = for {
          shift-right: [w509] -> w394
          shift-left: refnum<vi>[] [] -> [w510]
          tunnel: w404 -> [w505] mode=indexing
          shift-right: [w508] -> w396
          shift-left: path "" -> [w503]
          shift-right: [w501] -> w387
          shift-left: i32[] [] -> [w500]
          i -> [w502]
          n131 = property class="LVClassLibrary"(reference=w505) -> ("Path"=w504:path)  [unwired: 1 in, 2 out]
          n132 = Path to Array of Strings(0:w504) -> (2:w507:string[])  [unwired: 1 out]
          n133 = To Lower Case(string=w507) -> (all lower case string=w512:string[])
          n134 = Search 1D Array(1D array=w512, element="messages") -> (index of element=w506:i32)  [unwired: 1 in]
          n135 = Greater Or Equal To 0?(x=w506) -> (x >= 0?=w511:bool)
          n136 = case shown="True" w511 {
            tunnel: w510 -> [w516 w526]
            tunnel: w505 -> [_ w525]
            tunnel: [w516 w524] -> w509
            tunnel: w503 -> [w515 _]
            tunnel: [w515 w521] -> w508
            tunnel: w507 -> [_ w523]
            tunnel: w506 -> [_ w520]
            tunnel: w502 -> [_ w517]
            tunnel: w500 -> [w514 w518]
            tunnel: [w514 w519] -> w501
            frame False {
            }
            frame True {
              n137 = Build Array (concatenate)(w526, w525) -> (w524:refnum<vi>[])
              n138 = Build Array (concatenate)(w518, w517) -> (w519:i32[])
              n139 = Array Subset(array=w523, length=w520) -> (w522:string[])  [unwired: 1 in]
              n140 = Array of Strings to Path(0:w522) -> (2:w521:path)  [unwired: 1 in]
            }
          }
        }
        n141 = for {
          shift-right: [w489] -> w392
          shift-left: refnum<vi>[] [] -> [w490]
          tunnel: w402 -> [w488] mode=indexing
          n142 = property class="VI"(reference=w488) -> ("Path"=w487:path)  [unwired: 1 in, 2 out]
          n143 = Path to Array of Strings(0:w487) -> (2:w495:string[])  [unwired: 1 out]
          n144 = To Lower Case(string=w495) -> (all lower case string=w493:string[])
          n145 = Search 1D Array(1D array=w493, element="messages") -> (index of element=w492:i32)  [unwired: 1 in]
          n146 = Greater Or Equal To 0?(x=w492) -> (x >= 0?=w491:bool)
          n147 = case shown="True" w491 {
            tunnel: w490 -> [w496 w499]
            tunnel: [w496 w498] -> w489
            tunnel: w488 -> [_ w497]
            frame False {
            }
            frame True {
              n148 = Build Array (concatenate)(w499, w497) -> (w498:refnum<vi>[])
            }
          }
        }
        n149 = Array Size(array=w394) -> (size(s)=w397:i32)
        n150 = case shown="1.." w397 {
          tunnel: w396 -> [_ w438]
          tunnel: w395 -> [_ w427]
          tunnel: w394 -> [_ w442]
          tunnel: w393 -> [w407 w441]
          tunnel: w392 -> [_ w440]
          tunnel: w391 -> [_ w434]
          tunnel: w390 -> [_ w431]
          tunnel: [w407 w417] -> w389
          tunnel: w387 -> [_ w416]
          tunnel: w386 -> [_ w415]
          tunnel: w385 -> [w406 w414]
          tunnel: [w406 w413] -> w384
          frame 0, Default {
          }
          frame 1.. {
            n151 = Build Path(base path=w438, name or relative path=w427) -> (appended path=w444:path)
            n152 = Build Path(base path=w438, name or relative path="Messages" ("element")) -> (appended path=w435:path)
            n153 = To Lower Case(string=w434) -> (all lower case string=w433:string[])
            n154 = call <resource>:"File_CreateFolders.vi"("Path"=w444, "error in (no error)"=w441) -> ("error out"=w443:errorcluster)  [unwired: 15 in, 2 out]
            n155 = Search 1D Array(1D array=w433, element="messages") -> (index of element=w430:i32)  [unwired: 1 in]
            n156 = for {
              tunnel: w444 -> [_]
              tunnel: w442 -> [w486] mode=indexing
              tunnel: w427 -> [w480]
              shift-right: [w473] -> w439
              shift-left: w443 -> [w478]
              tunnel: [w472] -> w418 mode=indexing
              n157 = property class="LVClassLibrary"(reference=w486, error in=w478) -> (reference out=w479:refnum<vi>, error out=w475:errorcluster, "Path"=w483:path)
              n158 = Path to Array of Strings(0:w483) -> (2:w482:string[])  [unwired: 1 out]
              n159 = To Lower Case(string=w482) -> (all lower case string=w485:string[])
              n160 = Search 1D Array(1D array=w485, element="messages") -> (index of element=w481:i32)  [unwired: 1 in]
              n161 = Replace Array Subset(array=w482, new element=w480, index=w481) -> (w477:string[])
              n162 = Array of Strings to Path(0:w477) -> (2:w472:path)  [unwired: 1 in]
              n163 = Strip Path(path=w472) -> (stripped path=w476:path)  [unwired: 1 out]
              n164 = call <resource>:"File_CreateFolders.vi"("Path"=w476, "error in (no error)"=w475) -> ("error out"=w474:errorcluster)  [unwired: 15 in, 2 out]
              n165 = invoke class="LVClassLibrary" method="Save"(reference=w479, error in=w474, "Path"=w472) -> (error out=w473:errorcluster)  [unwired: 1 in, 3 out]
            }
            n166 = for {
              tunnel: w440 -> [w471] mode=indexing
              tunnel: w427 -> [w465]
              shift-right: [w457] -> w436
              shift-left: w439 -> [w463]
              n167 = property class="VI"(reference=w471, error in=w463) -> (reference out=w464:refnum<vi>, error out=w460:errorcluster, "Path"=w468:path)
              n168 = Path to Array of Strings(0:w468) -> (2:w467:string[])  [unwired: 1 out]
              n169 = To Lower Case(string=w467) -> (all lower case string=w470:string[])
              n170 = Search 1D Array(1D array=w470, element="messages") -> (index of element=w466:i32)  [unwired: 1 in]
              n171 = Replace Array Subset(array=w467, new element=w465, index=w466) -> (w462:string[])
              n172 = Array of Strings to Path(0:w462) -> (2:w458:path)  [unwired: 1 in]
              n173 = Strip Path(path=w458) -> (stripped path=w461:path)  [unwired: 1 out]
              n174 = call <resource>:"File_CreateFolders.vi"("Path"=w461, "error in (no error)"=w460) -> ("error out"=w459:errorcluster)  [unwired: 15 in, 2 out]
              n175 = invoke class="VI" method="Save.Instrument"(reference=w464, error in=w459, "Path to saved file"=w458) -> (error out=w457:errorcluster)  [unwired: 3 in, 5 out]
            }
            n176 = Index Array(array=w431, index=w430) -> (element=w429:refnum<vi>)
            n177 = Delete(path (use dialog)=w435, entire hierarchy (F)=TRUE, error in=w436) -> (error out=w424:errorcluster)  [unwired: 2 in, 2 out]
            n178 = property class="ProjectItem"(reference=w429, error in=w424) -> (reference out=w422:refnum<vi>, error out=w423:errorcluster, "Parent"=w428:refnum<vi>)
            n179 = invoke class="ProjectItem" method="AddItem"(reference=w428, error in=w423, "Name"=w427, "Path"=path "", "Type"="Folder") -> (reference out=w408:refnum<vi>, error out=w420:errorcluster, "AddItem"=w409:refnum<vi>)  [unwired: 1 in, 3 out]
            n180 = invoke class="ProjectItem" method="Delete"(reference=w422, error in=w420) -> (error out=w419:errorcluster)  [unwired: 1 in, 2 out]
            n181 = for {
              tunnel: w409 -> [w456]
              tunnel: w418 -> [w454] mode=indexing
              shift-right: [w451] -> w410
              shift-left: w419 -> [w455]
              shift-right: [w449] -> w412
              shift-left: w415 -> [w447]
              tunnel: w416 -> [w446] mode=indexing
              tunnel: [w445] -> w411 mode=indexing
              n182 = invoke class="ProjectItem" method="AddFile"(reference=w456, error in=w455, "Path"=w454) -> (error out=w453:errorcluster, "AddFile"=w450:refnum<vi>)  [unwired: 1 in, 2 out]
              n183 = Index Array(array=w447, index=w446) -> (element=w445:refnum<vi>)
              n184 = To More Specific Class(target class=refnum<vi> refnum ("Library"), reference=w450, error in=w453) -> (specific class reference=w448:refnum<vi>, error out=w451:errorcluster)
              n185 = Replace Array Subset(array=w447, new element=w448, index=w446) -> (w449:refnum<vi>[])
            }
            n186 = Bundle By Name(cluster=w414, "LibraryClasses"=w412) -> (w413:T2)
            n187 = Close Reference(reference=w409, error in (no error)=w410) -> (error out=w417:errorcluster)
            n188 = Close Reference(reference=w411) -> ()  [unwired: 1 in, 1 out]
            n189 = Close Reference(reference=w408, error in (no error)=w410) -> ()  [unwired: 1 out]
          }
        }
      }
      frame "UpdateClassProperties" {
        n190 = Unbundle By Name(w533) -> ("LibraryClasses"=w539:refnum<vi>[], "ClassTemplateVersion"=w537:string, "ClassesRootClass"=w536:string[])
        n191 = Variant To Data(type=path "" ("Path"), Variant=w529) -> (data=w530:path, error out=w528:errorcluster)  [unwired: 1 in]
        n192 = Empty String/Path?(string/path=w530) -> (empty?=w527:bool)
        n193 = for {
          tunnel: w539 -> [w557] mode=indexing
          tunnel: T3 {"ClassProviderName"="", "ClassTemplateUsed"="", "ClassTemplateVersion"="", "ClassDescription"="", "PlugIns"=[], "ConnectorPanePattern"=""} ("ClassSettings") -> [w577]
          tunnel: w541 -> [w575]
          tunnel: w540 -> [w574]
          shift-right: [w555] -> w535
          shift-left: w542 -> [w569]
          tunnel: w538 -> [w573]
          tunnel: w537 -> [w572]
          tunnel: w536 -> [w559] mode=indexing
          tunnel: [w551] -> w534 mode=indexing
          tunnel: w528 -> [_]
          tunnel: w527 -> [w550]
          w556 = T10 0 items=["4x4x4", "5x6x5", "6x8x6"] ("PatternOut")
          n194 = Match Pattern(string=w559, regular expression="\\2E[Ll][Vv][Cc][Ll][Aa][Ss][Ss]$") -> (before substring=w558:string)  [unwired: 1 in, 3 out]
          n195 = To Lower Case(string=w558) -> (all lower case string=w565:string)
          n196 = Equal?(x=w565, y="message") -> (x = y?=w548:bool)
          n197 = Select(t=u8 3 ("HeaderRows(1)"), s=w548, f=u8 0 ("HeaderRows(1)")) -> (s? t:f=w563:u8)
          n198 = Bundle By Name(cluster=T7 {"LibraryIcon"="Normal", "HeaderRows(1)"=0} ("LibraryIcon"), "LibraryIcon"=w558, "HeaderRows(1)"=w563) -> (w567:T7)
          n199 = call <resource>:"GDSLvIcon_DialogUpdateClass.vi"("ClassPath(FilePath/ProjectTreePath/LvCLassRef)"=w557, "AutoUpdate"=TRUE, "error in (no error)"=w569, "LibraryIcon"=w567) -> ("error out"=w554:errorcluster)  [unwired: 12 in, 3 out]
          n200 = Compound Arithmetic op=AND(invert w548, invert w550) -> (w551:bool)
          n201 = Format Into String(w556) -> (resulting string=w549:string)  [unwired: 3 in, 1 out]
          n202 = Select(t=ClassApperanceType."AF-MessageClass" ("ClassType(Class)"), s=w548, f=ClassApperanceType."Class" ("ClassType(Class)")) -> (s? t:f=w547:T6)
          n203 = Bundle By Name(cluster=w577, "ClassProviderName"=w575, "ClassTemplateUsed"=w573, "ClassTemplateVersion"=w572, "ClassDescription"=w574, "ConnectorPanePattern"=w549) -> (w576:T3)
          n204 = call <resource>:"GDSLvClass_StoreClassType.vi"("Class Refnum In"=w557, "ClassSettings"=w576, "error in (no error)"=w554) -> ("Class Refnum Out"=w571:refnum<vi>, "error out"=w570:errorcluster)  [unwired: 15 in]
          n205 = call <resource>:"UpdateClassApperance.vi"("ClassRefIn"=w571, "ClassType(Class)"=w547, "error in (no error)"=w570) -> ("ClassRefOut"=w553:refnum<vi>, "error out"=w552:errorcluster)  [unwired: 15 in]
          n206 = disable-structure shown="Enabled" {
            disable-tunnel: [w581 w582] -> w555
            disable-tunnel: w553 -> [w580 _]
            disable-tunnel: w552 -> [w579 w582]
            frame Disabled {
              n207 = invoke class="LVClassLibrary" method="Save"(reference=w580, error in=w579) -> (error out=w578:errorcluster)  [unwired: 2 in, 3 out]
              n208 = call <resource>:"CommonVIs_Wait.vi"("error in"=w578) -> ("error out"=w581:errorcluster)  [unwired: 9 in]
            }
            frame Enabled {
            }
          }
        }
        n209 = Bundle By Name(cluster=w533, "AddInheritance"=w534) -> (w532:T2)
      }
      frame "AddLibraryToProject" {
        n210 = Unbundle By Name(w594) -> ("ProjectItemOwner"=w588:refnum<vi>, "lvlib"=w592:bool, "Library"=w601:refnum<vi>, "LibraryClasses"=w611:refnum<vi>[])
        n211 = Index Array(array=w611) -> (element=w600:refnum<vi>)  [unwired: 1 in]
        n212 = Select(t=w601, s=w592, f=w600) -> (s? t:f=w602:refnum<vi>)
        n213 = call <resource>:"GDSLvIcon_DialogUpdateClass.vi"("ClassPath(FilePath/ProjectTreePath/LvCLassRef)"=w602, "AutoUpdate"=TRUE, "error in (no error)"=w612) -> ("error out"=w603:errorcluster)  [unwired: 13 in, 3 out]
        n214 = flat-sequence {
          tunnel: w594 -> [w646]
          tunnel: w603 -> [w640]
          tunnel: [w644] -> w609
          tunnel: [w643] -> w608
          tunnel: [w642] -> w599
          tunnel: [w637] -> w596
          tunnel: [w638] -> w595
          tunnel: w592 -> [w661]
          tunnel: w601 -> [w660]
          tunnel: w609 -> [w659]
          tunnel: w608 -> [w658]
          tunnel: [w652] -> w607
          tunnel: [w656] -> w606
          tunnel: [w655] -> w605
          tunnel: [w657] -> w604
          tunnel: w596 -> [w653]
          tunnel: [w651] -> w590
          tunnel: w607 -> [w674]
          tunnel: w606 -> [w677]
          tunnel: w605 -> [w676]
          tunnel: w604 -> [w675]
          tunnel: [w674] -> w589
          tunnel: [w671] -> w591
          tunnel: w590 -> [w671]
          frame #0 {
            n215 = Unbundle By Name(w646) -> ("FolderItems"=w645:refnum<vi>[], "LibraryClasses"=w643:refnum<vi>[], "LibraryVIs"=w644:refnum<vi>[])
            n216 = call <resource>:"GOOP_DebugLogger.vi"("error in (no error)"=w640, "State"="Save Case 1") -> ("error out"=w639:errorcluster)  [unwired: 7 in, 2 out]
            n217 = stacked-sequence {
              tunnel: w645 -> [w648]
              tunnel: [w647] -> w637
              tunnel: w639 -> [w647]
              frame #0 {
                n218 = Close Reference(reference=w648) -> ()  [unwired: 1 in, 1 out]
              }
            }
            n219 = for {
              tunnel: w643 -> [w650] mode=indexing
              tunnel: [w649] -> w638 mode=indexing
              n220 = property class="LVClassLibrary"(reference=w650) -> ("Path"=w649:path)  [unwired: 1 in, 2 out]
            }
            n221 = Index Array(array=w638) -> (element=w642:path)  [unwired: 1 in]
          }
          frame #1 {
            n222 = call <resource>:"GOOP_DebugLogger.vi"("error in (no error)"=w653, "State"="Save Case 2") -> ("error out"=w652:errorcluster)  [unwired: 7 in, 2 out]
            n223 = case shown="True" w661 {
              tunnel: w660 -> [_ w670]
              tunnel: [_ w667] -> w656
              tunnel: w652 -> [_ _]
              tunnel: [_ w666] -> w651
              frame False {
              }
              frame True {
                n224 = invoke class="Library" method="Save"(reference=w670) -> (reference out=w669:refnum<vi>, error out=w668:errorcluster)  [unwired: 3 in, 2 out]
                n225 = property class="Library"(reference=w669, error in=w668) -> (reference out=w667:refnum<vi>, "Path"=w666:path)  [unwired: 1 out]
              }
            }
            n226 = for {
              tunnel: w658 -> [w665] mode=indexing
              tunnel: [w664] -> w655 mode=indexing
              tunnel: w656 -> [_]
              n227 = invoke class="LVClassLibrary" method="Save"(reference=w665) -> (reference out=w664:refnum<vi>)  [unwired: 3 in, 3 out]
            }
            n228 = for {
              tunnel: w659 -> [w663] mode=indexing
              tunnel: [w662] -> w657 mode=indexing
              tunnel: w655 -> [_]
              n229 = invoke class="VI" method="Save.Instrument"(reference=w663) -> (reference out=w662:refnum<vi>)  [unwired: 5 in, 5 out]
            }
          }
          frame #2 {
            n230 = Close Reference(reference=w677) -> (error out=w673:errorcluster)  [unwired: 1 in]
            n231 = Close Reference(reference=w676, error in (no error)=w673) -> (error out=w672:errorcluster)
            n232 = Close Reference(reference=w675, error in (no error)=w672) -> ()  [unwired: 1 out]
          }
        }
        n233 = Bundle By Name(cluster=w594, "LibraryClasses(Path)"=w595) -> (w593:T2)
        n234 = property class="ProjectItem"(reference=w588) -> (reference out=w587:refnum<vi>, "Connected to Disk"=w586:path)  [unwired: 1 in, 1 out]
        n235 = Empty String/Path?(string/path=w586) -> (empty?=w584:bool)
        n236 = Not A Number/Path/Refnum?(number/path/refnum=w586) -> (NaN/Path/Refnum?=w585:bool)
        n237 = Or(x=w584, y=w585) -> (x .or. y?=w583:bool)
        n238 = case shown="False" w583 {
          tunnel: w599 -> [_ w620]
          tunnel: [w614 w619] -> w598
          tunnel: w592 -> [_ w618]
          tunnel: w591 -> [_ w617]
          tunnel: w589 -> [w614 w616]
          tunnel: w587 -> [_ w615]
          frame False {
          }
          frame True {
            n239 = case shown="True" w618 {
              tunnel: w615 -> [w629 w636]
              tunnel: [w621 w635] -> w619
              tunnel: w616 -> [w626 w633]
              tunnel: w620 -> [_ w631]
              tunnel: w617 -> [w624 _]
              frame True {
                n240 = Path To String(path=w624) -> (string=w627:string)
                n241 = call <resource>:"GOOP_DebugLogger.vi"("error in (no error)"=w626, "Data"=w627, "State"="TimeToAdd") -> ("error out"=w625:errorcluster)  [unwired: 6 in, 2 out]
                n242 = invoke class="ProjectItem" method="AddFile"(reference=w629, error in=w625, "Path"=w624) -> (error out=w622:errorcluster)  [unwired: 1 in, 3 out]
                n243 = call <resource>:"GDSError_ClearError.vi"("codes"=i32[] [56002], "error in (no error)"=w622) -> ("error out"=w621:errorcluster)  [unwired: 16 in, 1 out]
              }
              frame False {
                n244 = Path To String(path=w631) -> (string=w630:string)
                n245 = call <resource>:"GOOP_DebugLogger.vi"("error in (no error)"=w633, "Data"=w630, "State"="TimeToAdd") -> ("error out"=w632:errorcluster)  [unwired: 6 in, 2 out]
                n246 = invoke class="ProjectItem" method="AddFile"(reference=w636, error in=w632, "Path"=w631) -> (error out=w635:errorcluster)  [unwired: 1 in, 3 out]
              }
            }
          }
        }
        n247 = call <resource>:"CommonVIs_Wait.vi"("error in"=w598) -> ("error out"=w597:errorcluster)  [unwired: 9 in]
      }
      frame "SetInheritance" {
        n248 = Unbundle By Name(w685) -> ("AddInheritance"=w682:bool[], "LibraryClasses(Path)"=w679:path[], "App"=w678:refnum<vi>)
        n249 = Search 1D Array(1D array=w682, element=TRUE) -> (index of element=w680:i32)  [unwired: 1 in]
        n250 = case shown="Default" w680 {
          selector: w680 -> [w700 _]
          tunnel: w679 -> [w701 _]
          tunnel: w678 -> [w699 _]
          tunnel: w687 -> [w695 w705]
          tunnel: w683 -> [w694 _]
          tunnel: [w688 w705] -> w686
          frame Default {
            n251 = Index Array(array=w701, index=w700) -> (element=w698:path)
            n252 = invoke class="App" method="LVClass.Open"(reference=w699, error in=w695, "Path"=w698) -> (error out=w696:errorcluster, "LVClass.Open"=w697:refnum<vi>)  [unwired: 1 in, 2 out]
            n253 = call <resource>:"GDSProject_OpenClass.vi"("ClassPath(FilePath/ProjectTreePath/LvCLassRef)"=w694, "error IO"=w696) -> ("LVClass.Open"=w691:refnum<vi>, "error out"=w693:errorcluster)  [unwired: 15 in, 1 out]
            n254 = property class="LVClassLibrary"(reference=w697, error in=w693, "Parent"=w691) -> (reference out=w692:refnum<vi>, error out=w689:errorcluster)
            n255 = invoke class="LVClassLibrary" method="Save"(reference=w692, error in=w689) -> (reference out=w690:refnum<vi>, error out=w688:errorcluster)  [unwired: 2 in, 2 out]
            n256 = stacked-sequence {
              tunnel: w691 -> [w704]
              tunnel: w690 -> [w703]
              tunnel: w688 -> [_]
              frame #0 {
                n257 = Close Reference(reference=w704) -> (error out=w702:errorcluster)  [unwired: 1 in]
                n258 = Close Reference(reference=w703, error in (no error)=w702) -> ()  [unwired: 1 out]
              }
            }
          }
          frame -1 {
          }
        }
      }
      frame "Error", "Exit", Default {
        n259 = call <resource>:"GDSError_LogErrorInformation.vi"("State"=w707, "LocalVariableData"=w706, "error in (no error)"=w709) -> ("error out"=w708:errorcluster)  [unwired: 16 in]
      }
    }
    n260 = Select(t="Error", s=w33, f=w32) -> (s? t:f=w31:string)
  }
  "error out" <- w18
  n261 = Unbundle By Name(w12) -> ("App"=w10:refnum<vi>, "ProjectRefnum"=w5:refnum<vi>, "DestroyProjectItemRef"=w2:bool, "ProjectItemOwner"=w7:refnum<vi>)
  n262 = Unbundle By Name(w12) -> ()  [unwired: 1 out]
  n263 = call <resource>:"GOOP_DebugLogger.vi"("State"=w9) -> ("error out"=w8:errorcluster)  [unwired: 8 in, 2 out]
  n264 = Close Reference(reference=w10, error in (no error)=w8) -> (error out=w4:errorcluster)
  n265 = Close Reference(reference=w5, error in (no error)=w4) -> (error out=w3:errorcluster)
  n266 = stacked-sequence {
    tunnel: w7 -> [w715]
    tunnel: w3 -> [w714]
    tunnel: [refnum<vi> refnum ("LVClassLibraryRefnum")] -> w6
    tunnel: w2 -> [w712]
    frame #0 {
      n267 = case shown="True" w712 {
        tunnel: w715 -> [_ w717]
        tunnel: w714 -> [_ w716]
        frame False {
        }
        frame True {
          n268 = Close Reference(reference=w717, error in (no error)=w716) -> ()  [unwired: 1 out]
        }
      }
    }
  }
  "LVClassLibraryRefnum" <- w6
